vi "CheckProjectConditionalDeactivationValues.vi"(7 "Datei erstellen":bool, 8 "Fehler (Eingang, kein Fehler)":errorcluster, 9 "Value aus Datei":string[](array[string]), 10 "Key aus Datei":string[](array[string]), 11 "Project Path":path) -> (0 "Fehler (Ausgang)":errorcluster, 3 "Project Path out":path)   [LabVIEW 2020, in "ConditionalDeactivation.lvlib"]
uses:
  ConditionalDeactivation.lvlib
  <vilib>/Utility/file.llb/Write Delimited Spreadsheet (string).vi
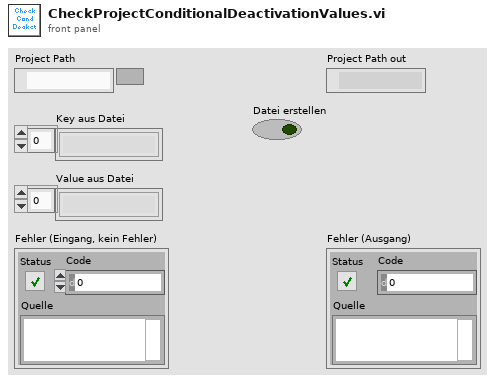
[diagram p1: front panel]
types:
  T1 = cluster{"Key aus Datei":string[], "Value aus Datei":string[]}
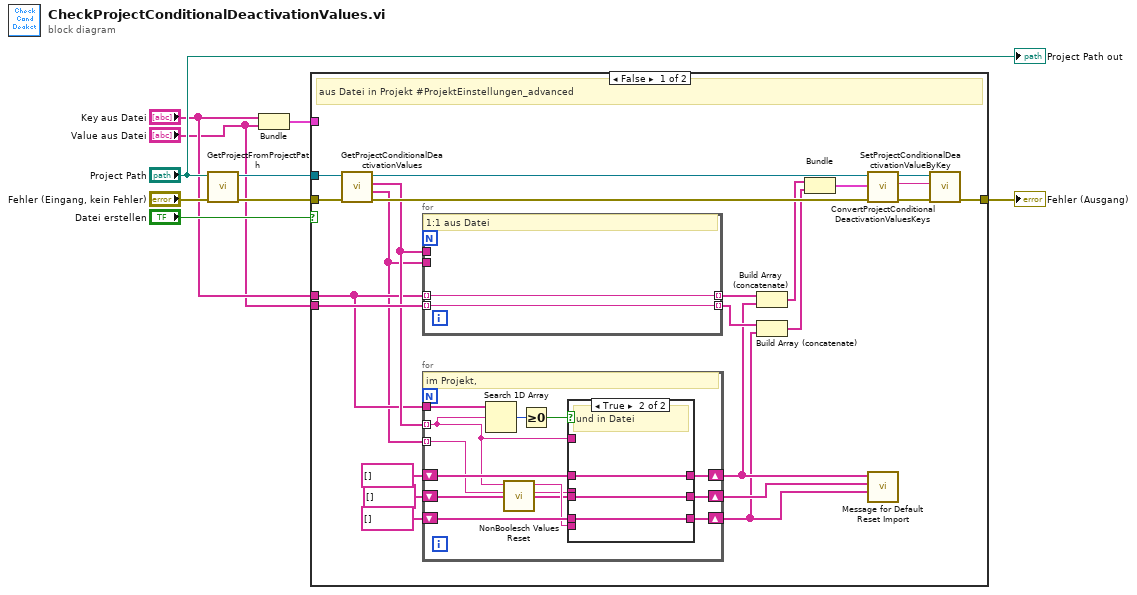
[diagram p0: block diagram]
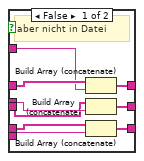
[diagram p2: hidden frame]
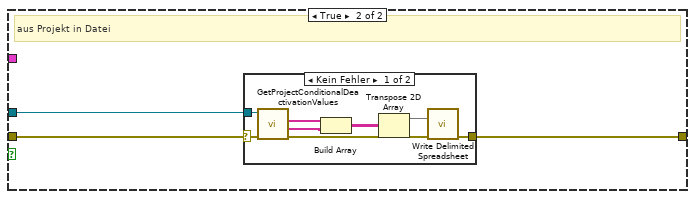
[diagram p3: hidden frame]
diagram:
  n1 = call "GetProjectFromProjectPath.vi"("Fehler (Eingang, kein Fehler)"="Fehler (Eingang, kein Fehler)", "ProjectPfad"="Project Path") -> ("Fehler (Ausgang)"=w9:errorcluster, "Projekt Referenz"=w4:refnum<vi>)  [unwired: 8 in]
  n2 = Bundle("Key aus Datei"="Key aus Datei", "Value aus Datei"="Value aus Datei") -> (w1:T1)  [unwired: 1 in]
  n3 = case shown="False" "Datei erstellen" {
    tunnel: w9 -> [w30 w58]
    tunnel: w1 -> [_ _]
    tunnel: [w27 w59] -> w6
    tunnel: w4 -> [w26 w60]
    tunnel: "Key aus Datei" -> [w22 _]
    tunnel: "Value aus Datei" -> [w24 _]
    frame False {
      # "aus Datei in Projekt #ProjektEinstellungen_advanced"
      n4 = call "GetProjectConditionalDeactivationValues.vi"("Projekt Referenz"=w26) -> ("Values aus Projekt"=w14:string[], "Keys aus Projekt"=w23:string[], "Projekt Referenz"=w25:refnum<vi>)  [unwired: 6 in, 2 out]
      n5 = for {
        tunnel: w22 -> [w57] mode=indexing
        tunnel: w23 -> [_]
        tunnel: w14 -> [_]
        tunnel: w24 -> [w56] mode=indexing
        tunnel: [w57] -> w21 mode=indexing
        tunnel: [w56] -> w20 mode=indexing
        # "1:1 aus Datei"
      }
      n6 = for {
        tunnel: w23 -> [w35] mode=indexing
        tunnel: w22 -> [w42]
        shift-right: [w39] -> w12
        shift-left: string[] [] -> [w40]
        shift-right: [w38] -> w10
        shift-left: string[] [] -> [w37]
        tunnel: w14 -> [w34] mode=indexing
        shift-right: [w32] -> w11
        shift-left: string[] [] -> [w31]
        # "im Projekt,"
        n7 = Search 1D Array(1D array=w42, element=w35) -> (index of element=w43:i32)  [unwired: 1 in]
        n8 = call "NonBoolesch Values Reset.vi"("Value aus Projekt"=w34, "Key aus Projekt"=w35) -> ("Value aus Projekt out"=w33:string, "Default Value"=w36:string)  [unwired: 8 in]
        n9 = Greater Or Equal To 0?(x=w43) -> (x >= 0?=w41:bool)
        n10 = case shown="True" w41 {
          tunnel: w35 -> [w51 _]
          tunnel: w36 -> [w49 _]
          tunnel: [w50 w55] -> w39
          tunnel: w40 -> [w52 w55]
          tunnel: [w48 w54] -> w38
          tunnel: w37 -> [w47 w54]
          tunnel: w33 -> [w45 _]
          tunnel: [w46 w53] -> w32
          tunnel: w31 -> [w44 w53]
          frame False {
            # "aber nicht in Datei"
            n11 = Build Array (concatenate)(w52, w51) -> (w50:string[])
            n12 = Build Array (concatenate)(w44, w45) -> (w46:string[])
            n13 = Build Array (concatenate)(w47, w49) -> (w48:string[])
          }
          frame True {
            # "und in Datei"
          }
        }
      }
      n14 = Build Array (concatenate)(w21, w12) -> (w19:string[])
      n15 = Build Array (concatenate)(w20, w10) -> (w18:string[])
      n16 = Bundle(w19, w18) -> (w17:cluster{string[], string[]})  [unwired: 1 in]
      n17 = call "ConvertProjectConditionalDeactivationValuesKeys.vi"("Fehler (Eingang, kein Fehler)"=w30, "CondDeact"=w17) -> ("Fehler (Ausgang)"=w28:errorcluster, "Tabellen-String"=w29:string)  [unwired: 8 in]
      n18 = call "Message for Default Reset Import.vi"("New Value (Default)"=w10, "Old Value"=w11, "Key"=w12) -> ()  [unwired: 9 in]
      n19 = call "SetProjectConditionalDeactivationValueByKey.vi"("Fehler (Eingang, kein Fehler)"=w28, "Tabellen-String"=w29, "Projekt Referenz"=w25) -> ("Fehler (Ausgang)"=w27:errorcluster)  [unwired: 7 in, 1 out]
    }
    frame True {
      # "aus Projekt in Datei"
      n20 = case shown="Kein Fehler" w58 {
        selector: w58 -> [w62 w69]
        tunnel: w60 -> [w68 _]
        tunnel: [w64 w69] -> w59
        frame No Error {
          n21 = call "GetProjectConditionalDeactivationValues.vi"("Fehler (Eingang, kein Fehler)"=w62, "Projekt Referenz"=w68) -> ("Fehler (Ausgang)"=w61:errorcluster, "Values aus Projekt"=w65:string[], "Keys aus Projekt"=w66:string[])  [unwired: 5 in, 2 out]
          n22 = Build Array(w66, w65) -> (w67:string[][])
          n23 = Transpose 2D Array(2D array=w67) -> (transposed array=w63:string[][])
          n24 = call-poly <vilib>:"Write Delimited Spreadsheet.vi"("2D data"=w63, "error in (no error)"=w61) -> ("error out"=w64:errorcluster)  [unwired: 12 in, 1 out]
        }
        frame Error {
        }
      }
    }
  }
  "Fehler (Ausgang)" <- w6
  "Project Path out" <- "Project Path"
